vi "IMAQdx HL-Grab.vi"(8 "ErrIn":errorcluster, 11 "Camera":refnum<k21> caption="IMAQdx Session") -> (0 "ErrOut":errorcluster, 3 "ImgOut":T1)   [LabVIEW 2013]
doc: "Use this template to build a VI to use as a subVI."
uses:
  <vilib>/vision/Image Controls.llb/IMAQ Image.ctl
  <vilib>/vision/driver/NI_Vision_Acquisition_Software.lvlib
panel:
  in  "stop":bool
  out "Frame Rate":dbl(knob) scale=0.0..100.0
  # "Input Parameters"
  # "Output Parameters"
  # "VI Description:\nThis VI is created to Grab a image from imaging device."
  # ":: MVI Framework V1.0 ::\nAuthor:Gaoke Yang\nEmail: gaoke.yang@yahoo.com\nWeb: www.mvicontrol.com\nCopyright (C) 2013, MVI Technologies All Rights Reserved"
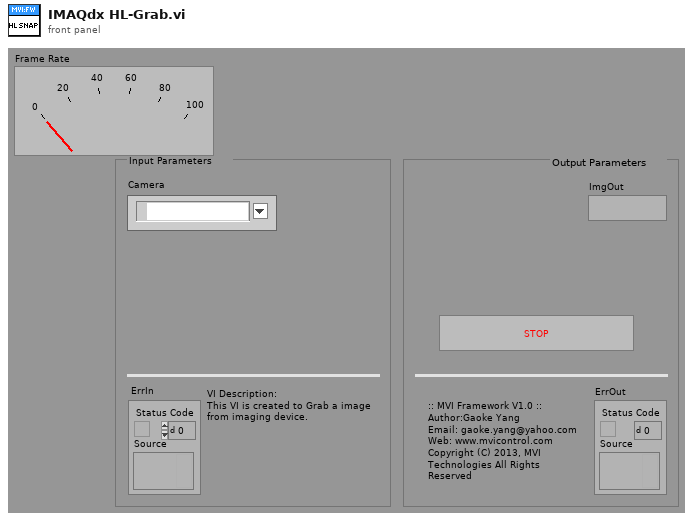
[diagram p1: front panel]
types:
  T1 = typedef "IMAQ Image.ctl" = refnum<image>
  T2 = typedef "IMAQdx.ctl" = refnum<k21>
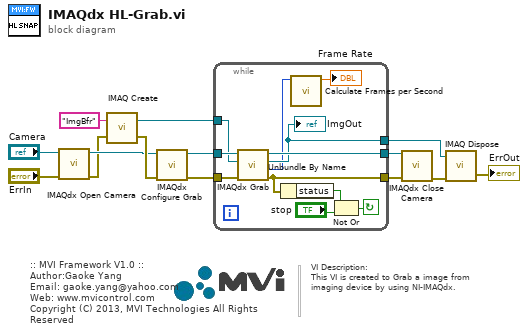
[diagram p0: block diagram]
diagram:
  # "VI Description:\nThis VI is created to Grab a image from \nimaging device by using NI-IMAQdx."
  # ":: MVI Framework V1.0 ::\nAuthor:Gaoke Yang\nEmail: gaoke.yang@yahoo.com\nWeb: www.mvicontrol.com\nCopyright (C) 2013, MVI Technologies All Rights Reserved"
  n1 = call <vilib>:"IMAQdx Open Camera.vi"("error in"="ErrIn", "Session In"="Camera") -> ("error out"=w1:errorcluster, "Session Out"=w2:T2)  [unwired: 8 in]
  n2 = call "IMAQ Create"("Image Name"="ImgBfr", "error in (no error)"=w1) -> ("New Image"=w10:T1, "error out"=w11:errorcluster)  [unwired: 2 in, 1 out]
  n3 = call <vilib>:"IMAQdx Configure Grab.vi"("error in"=w11, "Session In"=w2) -> ("error out"=w8:errorcluster, "Session Out"=w9:T2)  [unwired: 8 in]
  n4 = while {
    tunnel: [w19] -> w6
    tunnel: w10 -> [w23]
    tunnel: w9 -> [w24]
    tunnel: w8 -> [w25]
    tunnel: [w18] -> w5
    tunnel: [w17] -> w3
    stop <- w21 continue-if-true
    n5 = call <vilib>:"IMAQdx Grab.vi"("error in"=w25, "Image In"=w23, "Session In"=w24) -> ("error out"=w18:errorcluster, "Buffer Number Out"=w16:u32, "Image Out"=w17:T1, "Session Out"=w19:T2)  [unwired: 5 in]
    "ImgOut" <- w17
    n6 = Unbundle By Name(w18) -> ("status"=w22:bool)
    n7 = call <vilib>:"Calculate Frames per Second.vi"("Buffer Number"=w16) -> ("Acquired Frames/s"=→"Frame Rate":dbl)  [unwired: 8 in, 2 out]
    n8 = Not Or(1:"stop", 2:w22) -> (0:w21:bool)
  }
  n9 = call <vilib>:"IMAQdx Close Camera.vi"("error in"=w5, "Session In"=w6) -> ("error out"=w4:errorcluster)  [unwired: 9 in]
  n10 = call "IMAQ Dispose"("Image"=w3, "error in (no error)"=w4) -> ("error out"=→"ErrOut":errorcluster)  [unwired: 1 in, 3 out]
